vi "readreply.vi"(8 "error in (no error)":errorcluster, 9 "timeout ms (5000)":i32=5000, 10 "header chars (10)":i32=10, 11 "connection ID":refnum<k5>) -> (0 "error out":errorcluster, 3 "data out":string)   [LabVIEW 2015]
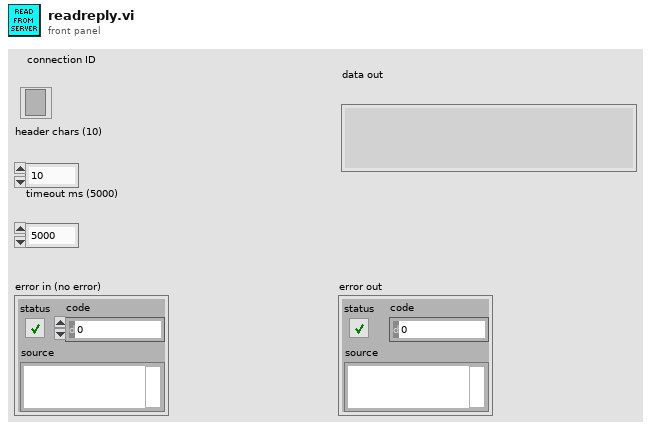
[diagram p1: front panel]
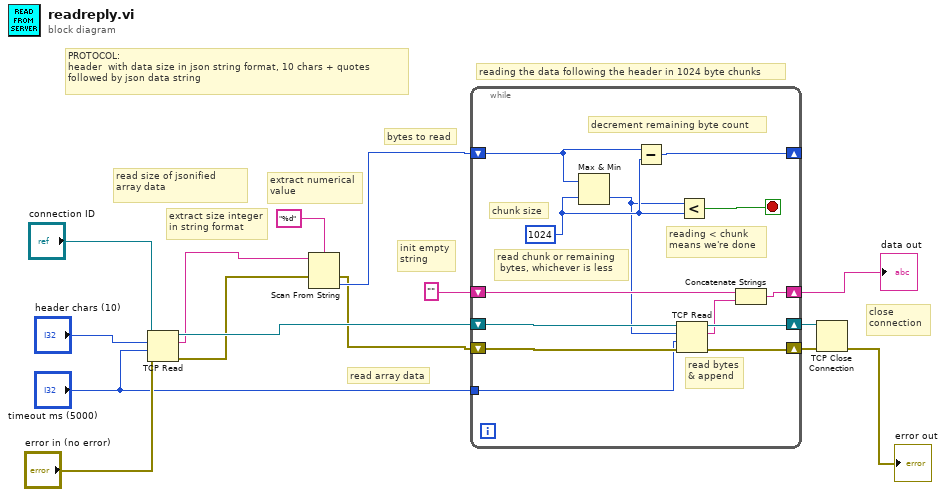
[diagram p0: block diagram]
diagram:
  # "PROTOCOL:\nheader  with data size in json string format, 10 chars + quotes \nfollowed by json data string"
  # "reading the data following the header in 1024 byte chunks"
  # "extract numerical\nvalue"
  # "close \nconnection"
  # "init empty\nstring"
  # "bytes to read"
  # "read array data"
  # "extract size integer\nin string format"
  # "read size of jsonified\narray data"
  n1 = TCP Read(connection ID="connection ID", bytes to read="header chars (10)", error in (no error)="error in (no error)", 9:"timeout ms (5000)") -> (connection ID out=w15:refnum<k5>, data out=w1:string, error out=w2:errorcluster)  [unwired: 1 in]
  n2 = Scan From String(format string="%d", input string=w1, error in=w2) -> (error out=w3:errorcluster, output 1=w4:i32)  [unwired: 2 in, 2 out]
  n3 = while {
    shift-right: [w25] -> w13
    shift-left: w3 -> [w28]
    shift-right: [w26] -> w14
    shift-left: w15 -> [w27]
    shift-right: [w24] -> _
    shift-left: w4 -> [w19]
    shift-right: [w21] -> w8
    shift-left: "" ("data out") -> [w23]
    tunnel: "timeout ms (5000)" -> [w20]
    stop <- w18 stop-if-true
    w17 = 1024
    # "read bytes\n& append"
    # "reading < chunk\nmeans we're done"
    # "decrement remaining byte count"
    # "read chunk or remaining\n bytes, whichever is less"
    # "chunk size"
    n4 = Max & Min(x=w19, y=w17) -> (min(x,y)=w16:i32)  [unwired: 1 out]
    n5 = Subtract(x=w19, y=w17) -> (x-y=w24:i32)
    n6 = TCP Read(connection ID=w27, bytes to read=w16, error in (no error)=w28, 9:w20) -> (connection ID out=w26:refnum<k5>, data out=w22:string, error out=w25:errorcluster)  [unwired: 1 in]
    n7 = Less?(x=w16, y=w17) -> (x < y?=w18:bool)
    n8 = Concatenate Strings(w23, w22) -> (w21:string)
  }
  "data out" <- w8
  n9 = TCP Close Connection(connection ID=w14, error in (no error)=w13) -> (error out=→"error out":errorcluster)  [unwired: 1 in, 1 out]
